vi "calcLoadCellExcitation.vi"(8 "error in (no error)":errorcluster, 10 "Reference Voltage Vref":dbl[unit] min=-10.0 max=10.0 format="%.3f", 11 "ForceSensor in":refnum<class "ForceSensor.lvclass">) -> (0 "error out":errorcluster, 3 "ForceSensor out":refnum<class "ForceSensor.lvclass">)   [LabVIEW 2013, in "ForceSensor.lvclass"]
uses:
  ForceSensor.lvclass
  ForceSensor.lvclass/ForceSensor.ctl
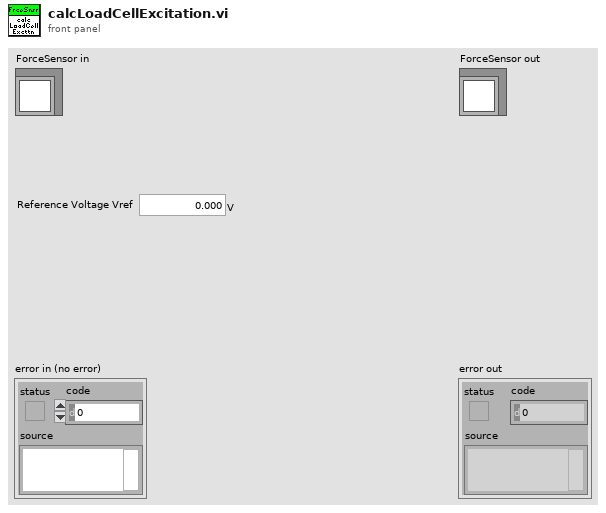
[diagram p1: front panel]
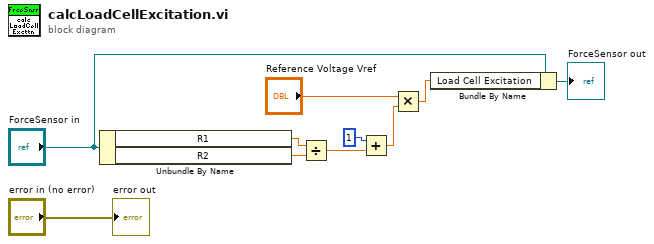
[diagram p0: block diagram]
diagram:
  n1 = Unbundle By Name("ForceSensor in") -> ("R1"=w6:dbl[unit], "R2"=w5:dbl[unit])
  n2 = Divide(x=w6, y=w5) -> (x/y=w4:dbl)
  n3 = Add(x=1, y=w4) -> (x+y=w3:dbl)
  n4 = Multiply(x="Reference Voltage Vref", y=w3) -> (x*y=w1:dbl[unit])
  n5 = Bundle By Name(cluster="ForceSensor in", "Load Cell Excitation"=w1) -> (→"ForceSensor out":refnum<class "ForceSensor.lvclass">)
  "error out" <- "error in (no error)"
